vi "Relink Export to userlib.vi"() -> ()   [LabVIEW 2020]
uses:
  Save for Previous Version.lvlib
  <userlib>/_OpenG.lib/file/file.llb/Build Path - File Names Array - path__ogtk.vi
  <userlib>/_OpenG.lib/file/file.llb/File Exists - Scalar__ogtk.vi
  <userlib>/_OpenG.lib/file/file.llb/Strip Path - Arrays__ogtk.vi
panel:
  out "Array 2":bool[](array[boolean])
  out "exists":bool[](array[boolean])
  out "Array":T1(array[cluster])
  in  "Target LabVIEW Installation":path
  out "error out 2":errorcluster
  out "Callers of user.lib":path[](array[path])
  out "Callers of user.lib":i32[](array[numeric])
  out "user.lib":i32[](array[numeric])
  out "New user.lib Paths":path[](array[path])
  in  "Source Folder":path
  in  "Listbox":i32(listbox)
  out "Linker Info out":T1(array[cluster])
  in  "Export Destination Folder":path
  out "error out":errorcluster
  in  "polys & tds":bool
  in  "recursive?":bool
  in  "paths to read":path[](array[path])
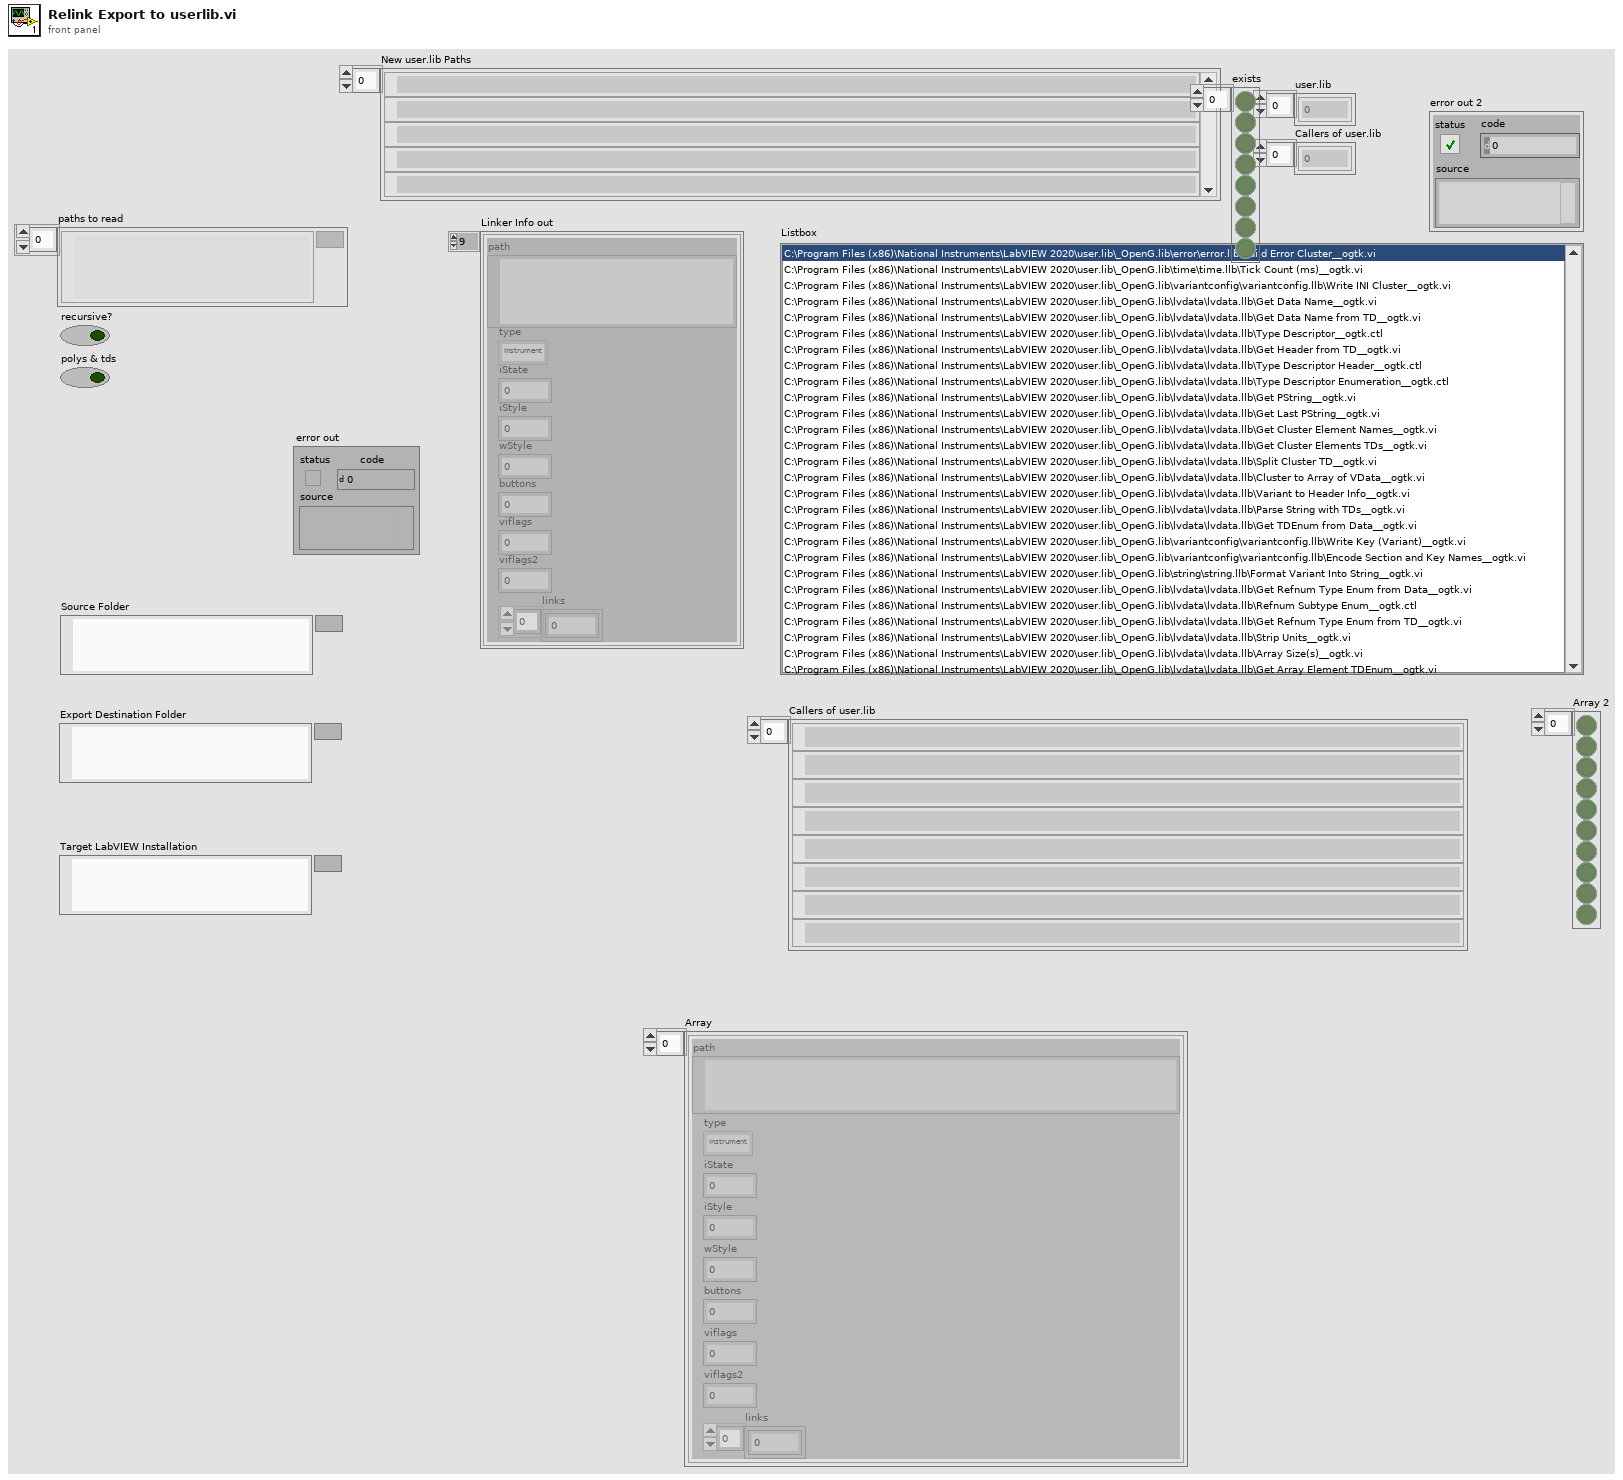
[diagram p1: front panel]
types:
  T1 = cluster{"path":path, "type":enum32{"Instrument", "Control", "CIN", "External subroutine", "Shared library", "Run-time menu", "Help file", "Palette menu"}, "iState":u32, "iStyle":u16, "wStyle":u16, "buttons":u16, "viflags":u32, "viflags2":u32, "links":u32[]}[]
  T2 = cluster{"path":path, "type":enum32{"Instrument", "Control", "CIN", "External subroutine", "Shared library", "Run-time menu", "Help file", "Palette menu"}, "iState":u32, "iStyle":u16, "wStyle":u16, "buttons":u16, "viflags":u32, "viflags2":u32, "links":u32[]}
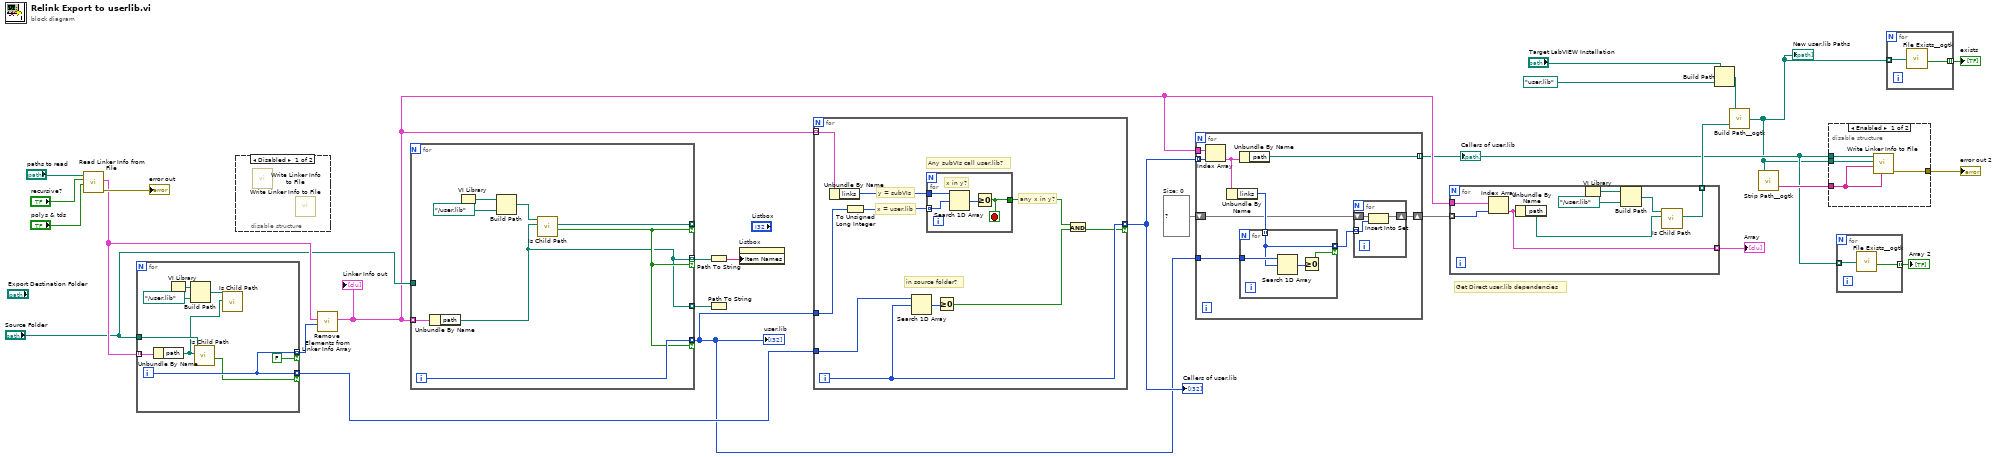
[diagram p0: block diagram]
diagram:
  w9 = set{u32} {}  # Size: 0
  # "Get Direct user.lib dependencies"
  n1 = call "Read Linker Info from File.vi"("polys & tds"="polys & tds", "recursive?"="recursive?", "paths to read"="paths to read") -> ("error out"=→"error out":errorcluster, "Read Linker Info from File"=w23:T1)  [unwired: 7 in]
  n2 = for {
    tunnel: w23 -> [w36] mode=indexing
    tunnel: "Source Folder" -> [w35]
    tunnel: [w29] -> w22 mode=indexing if=FALSE
    tunnel: [w29] -> w14 mode=indexing if=w28
    i -> [w29]
    n3 = Unbundle By Name(w36) -> ("path"=w31:path)
    n4 = VI Library() -> (path=w33:path)
    n5 = Build Path(base path=w33, name or relative path=path "../user.lib" ("path")) -> (appended path=w32:path)
    n6 = call "Is Child Path.vi"("File"=w31, "Base Folder"=w35) -> ("is Child Path"=w28:bool)  [unwired: 8 in, 1 out]
    n7 = call "Is Child Path.vi"("File"=w31, "Base Folder"=w32) -> ()  [unwired: 8 in, 2 out]
  }
  n8 = disable-structure shown="Disabled" {
    frame Disabled {
      n9 = call "Write Linker Info to File.vi"() -> ()  [unwired: 11 in, 1 out]
      n10 = call "Write Linker Info to File.vi"() -> ()  [unwired: 11 in, 1 out]
    }
    frame Enabled {
    }
  }
  n11 = call "Remove Elements from Linker Info Array.vi"("elements to remove"=w22, "Linker Info"=w23) -> ("Linker Info out"=w7:T1)  [unwired: 9 in]
  "Linker Info out" <- w7
  n12 = for {
    tunnel: w7 -> [w44] mode=indexing
    tunnel: "Source Folder" -> [_]
    tunnel: [w38] -> w21 mode=indexing
    tunnel: [w38] -> w20 mode=indexing if=w39
    tunnel: [w37] -> _ mode=indexing if=w39
    tunnel: [w40] -> w10 mode=indexing if=w39
    i -> [w40]
    n13 = Unbundle By Name(w44) -> ("path"=w38:path)
    n14 = VI Library() -> (path=w43:path)
    n15 = Build Path(base path=w43, name or relative path=path "../user.lib" ("path")) -> (appended path=w41:path)
    n16 = call "Is Child Path.vi"("File"=w38, "Base Folder"=w41) -> ("is Child Path"=w39:bool, "relative path from Base to File"=w37:path)  [unwired: 8 in]
  }
  "user.lib" <- w10
  n17 = Path To String(path=w20) -> (string=w19:string[])
  n18 = Path To String(path=w21) -> ()  [unwired: 1 out]
  n19 = property on="Listbox" class="LstBox (strict)"("Item Names"=w19) -> ()  [unwired: 2 in, 2 out]
  n20 = for {
    tunnel: w7 -> [w53] mode=indexing
    tunnel: [w48] -> w18 mode=indexing if=w47
    tunnel: w10 -> [w49]
    tunnel: w14 -> [w45]
    i -> [w48]
    # "in source folder?"
    # "any x in y?"
    # "Any subVIs call user.lib?"
    # "y = subVIs"
    # "x = user.lib"
    n21 = Unbundle By Name(w53) -> ("links"=w54:u32[])
    n22 = To Unsigned Long Integer(number=w49) -> (unsigned 32bit integer=w51:u32[])
    n23 = Search 1D Array(1D array=w45, element=w48) -> (index of element=w50:i32)  [unwired: 1 in]
    n24 = for {
      tunnel: w51 -> [w57] mode=indexing
      tunnel: w54 -> [w58]
      tunnel: [w55] -> w52
      stop <- w55 stop-if-true
      # "x in y?"
      n25 = Search 1D Array(1D array=w58, element=w57) -> (index of element=w56:i32)  [unwired: 1 in]
      n26 = Greater Or Equal To 0?(x=w56) -> (x >= 0?=w55:bool)
    }
    n27 = Greater Or Equal To 0?(x=w50) -> (x >= 0?=w46:bool)
    n28 = And(x=w52, y=w46) -> (x .and. y?=w47:bool)
  }
  "Callers of user.lib" <- w18
  n29 = for {
    tunnel: w18 -> [w67] mode=indexing
    tunnel: w7 -> [w66]
    tunnel: [w65] -> w3 mode=indexing
    tunnel: w10 -> [w62]
    shift-right: [w61] -> w8
    shift-left: w9 -> [w59]
    n30 = Index Array(array=w66, index=w67) -> (element=w64:T2)
    n31 = Unbundle By Name(w64) -> ("links"=w63:u32[])
    n32 = Unbundle By Name(w64) -> ("path"=w65:path)
    n33 = for {
      tunnel: w63 -> [w72] mode=indexing
      tunnel: w62 -> [w73]
      tunnel: [w72] -> w60 mode=indexing if=w71
      n34 = Search 1D Array(1D array=w73, element=w72) -> (index of element=w74:i32)  [unwired: 1 in]
      n35 = Greater Or Equal To 0?(x=w74) -> (x >= 0?=w71:bool)
    }
    n36 = for {
      tunnel: w60 -> [w69] mode=indexing
      shift-right: [w70] -> w61
      shift-left: w59 -> [w68]
      n37 = Insert Into Set(10:w69, 11:w68) -> (3:w70:set{u32})  [unwired: 1 out]
    }
  }
  "Callers of user.lib" <- w3
  n38 = for {
    tunnel: w8 -> [w82] mode=indexing
    tunnel: w7 -> [w81]
    tunnel: [w75] -> w6 mode=indexing
    tunnel: [w80] -> w5 mode=indexing
    n39 = Index Array(array=w81, index=w82) -> (element=w80:T2)
    n40 = Unbundle By Name(w80) -> ("path"=w76:path)
    n41 = VI Library() -> (path=w79:path)
    n42 = Build Path(base path=w79, name or relative path=path "../user.lib" ("path")) -> (appended path=w77:path)
    n43 = call "Is Child Path.vi"("File"=w76, "Base Folder"=w77) -> ("relative path from Base to File"=w75:path)  [unwired: 8 in, 1 out]
  }
  "Array" <- w5
  n44 = Build Path(base path="Target LabVIEW Installation", name or relative path=path "user.lib") -> (appended path=w11:path)
  n45 = call-poly <userlib>:"Build Path__ogtk.vi"("name or relative path"=w6, "base path"=w11) -> ("appended path"=w1:path[])
  "New user.lib Paths" <- w1
  n46 = call-poly <userlib>:"Strip Path__ogtk.vi"("path"=w1) -> ("name"=w16:string[])  [unwired: 1 out]
  n47 = disable-structure shown="Enabled" {
    disable-tunnel: w3 -> [w86 _]
    disable-tunnel: w1 -> [w85 _]
    disable-tunnel: [w84 _] -> w17
    disable-tunnel: w16 -> [w83 _]
    frame Enabled {
      n48 = call "Write Linker Info to File.vi"("New Names"=w83, "Old Names"=w83, "new paths"=w85, "files to change"=w86) -> ("error out"=w84:errorcluster)  [unwired: 7 in]
    }
    frame Disabled {
    }
  }
  "error out 2" <- w17
  n49 = for {
    tunnel: w3 -> [w88] mode=indexing
    tunnel: [w87] -> w2 mode=indexing
    n50 = call-poly <userlib>:"File Exists__ogtk.vi"("file path"=w88) -> ("exists"=w87:bool)  [unwired: 6 in, 1 out]
  }
  "Array 2" <- w2
  n51 = for {
    tunnel: w1 -> [w90] mode=indexing
    tunnel: [w89] -> w4 mode=indexing
    n52 = call-poly <userlib>:"File Exists__ogtk.vi"("file path"=w90) -> ("exists"=w89:bool)  [unwired: 6 in, 1 out]
  }
  "exists" <- w4
